vi "CubeDropper.vi"(1 "Shoot":bool, 2 "Height":enum16{"Switch", "Scale", "Bottom", "Null"}(ring)=enum."Scale") -> (0 "CurrentHeight":enum16{"Switch", "Scale", "Bottom", "Null"}(ring))   [LabVIEW 2017]
uses:
  <vilib>/Rock Robotics/WPI/ThirdParty/Phoenix-LabVIEW/Motor Controller/Controls/CTRE_Phoenix_MotorControl_ControlMode.ctl
  <vilib>/Rock Robotics/WPI/ThirdParty/Phoenix-LabVIEW/Motor Controller/Get/CTRE_Phoenix_MotorController_GetQuadratureData.vi
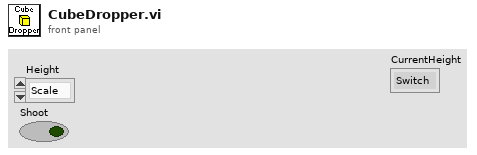
[diagram p1: front panel]
types:
  T1 = typedef "CTRE_Phoenix_MotorControl_ControlMode.ctl" = u16
  T2 = typedef "WPI_MotorControlDeviceRef.ctl" = cluster{"DeviceStatus":errorcluster, "Type":T3, "PWM":cluster{"PWM Channel":T4, "DeadBand":T5}, "CAN":cluster{"Device Number":u8, "SetOutput VI Ref":variant, "GetOutput VI Ref":variant, "Enable VI Ref":variant, "Disable VI Ref":variant, "Data":variant}, "Invert":bool, "DIO PWM":cluster{"PWM \"Enable\" Channel":T4, "DIOChannel":T6, "PWM Rate":dbl}}
  T3 = typedef "WPI_MotorControlType.ctl" = enum16{"PWM", "CAN", "DIO PWM"}
  T4 = typedef "FPGA_DIOPWMChannel.ctl" = enum8{"PWM 0", "PWM 1", "PWM 2", "PWM 3", "PWM 4", "PWM 5", "PWM 6", "PWM 7", "PWM 8", "PWM 9", "PWM MXP 0", "PWM MXP 1", "PWM MXP 2", "PWM MXP 3", "PWM MXP 4", "PWM MXP 5", "PWM MXP 6", "PWM MXP 7", "PWM MXP 8", "PWM MXP 9", "Invalid"}
  T5 = typedef "WPI_PWMDeadband.ctl" = cluster{"Name":string, "maxPositivePwm":i32, "minPositivePwm":i32, "centerPwm":i32, "maxNegativePwm":i32, "minNegativePwm":i32, "angularRange":u16}
  T6 = typedef "FPGA_DIOChannel.ctl" = enum8{"DIO 0", "DIO 1", "DIO 2", "DIO 3", "DIO 4", "DIO 5", "DIO 6", "DIO 7", "DIO 8", "DIO 9", "DIO MXP 0", "DIO MXP 1", "DIO MXP 2", "DIO MXP 3", "DIO MXP 4", "DIO MXP 5", "DIO MXP 6", "DIO MXP 7", "DIO MXP 8", "DIO MXP 9", "DIO MXP 10", "DIO MXP 11", "DIO MXP 12", "DIO MXP 13", "DIO MXP 14", "DIO MXP 15", "SPI Port CS1", "SPI Port CS2", "SPI Port CS3", "SPI Port MISO", "SPI Port MOSI", "Invalid"}
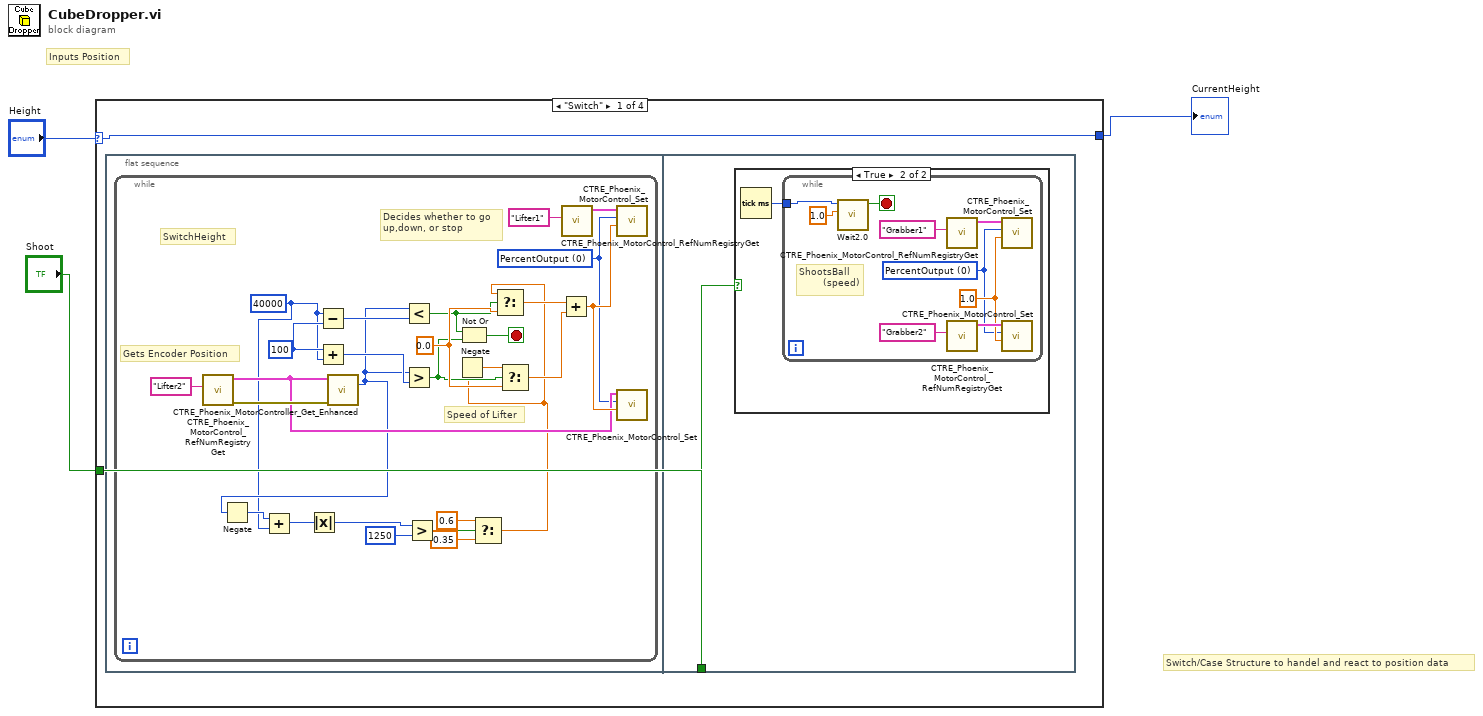
[diagram p0: block diagram]
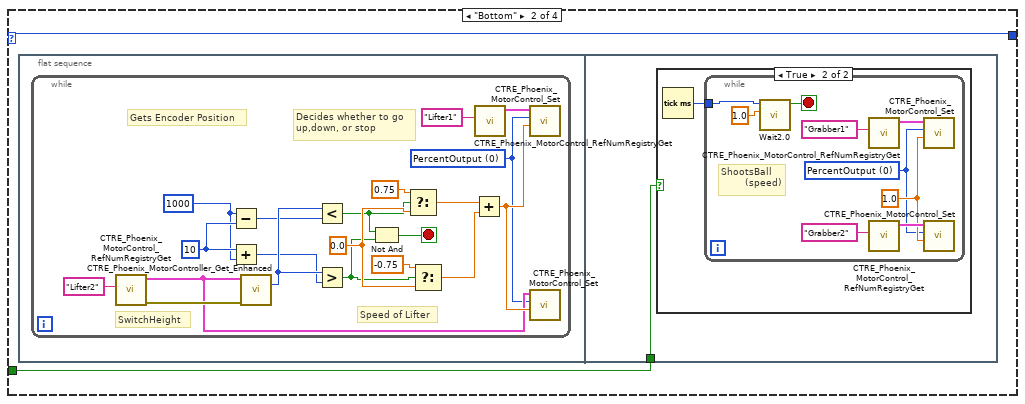
[diagram p3: hidden frame]
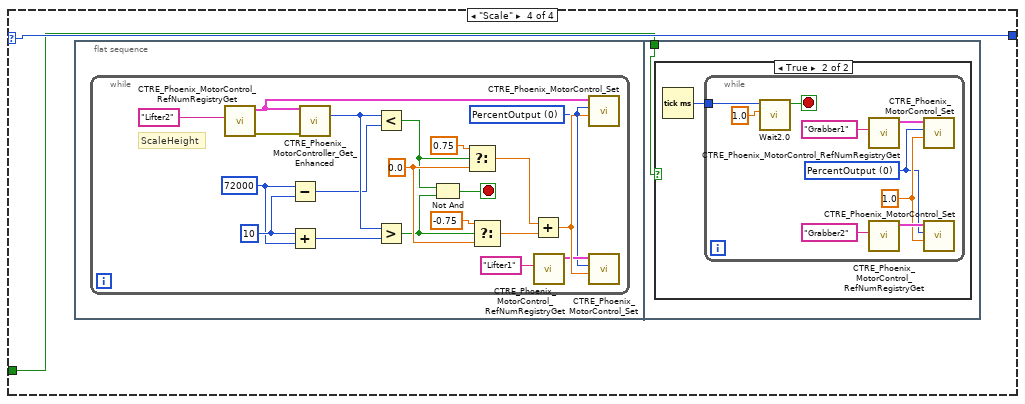
[diagram p6: hidden frame]
diagram:
  # "Switch/Case Structure to handel and react to position data"
  # "Inputs Position"
  n1 = case shown="\"Switch\"" "Height" {
    selector: "Height" -> [w5 w45 w77 w79]
    tunnel: [w5 w45 w77 w79] -> w2
    tunnel: "Shoot" -> [w4 w44 _ w78]
    frame "Switch" {
      n2 = flat-sequence {
        tunnel: w4 -> [w33]
        frame #0 {
          n3 = while {
            stop <- w21 stop-if-true
            w17 = T1 0 items=["PercentOutput"=0, "Position"=1, "Velocity"=2, "Current"=3, "Follower"=5, "MotionProfile"=6, "MotionMagic"=7, "MotionMagicArc"=8, "MotionProfileArc"=10, "Disabled"=15] ("Control Mode")
            w26 = 0.0
            w12 = 40000
            w29 = 100
            # "Speed of Lifter"
            # "Decides whether to go\nup,down, or stop"
            # "Gets Encoder Position"
            # "SwitchHeight"
            n4 = call <vilib>:"CTRE_Phoenix_MotorControl_RefNumRegistryGet.vi"("refnum name"="Lifter2") -> ("error out"=w32:errorcluster, "PhoenixMotorControlDevRef"=w19:T2)  [unwired: 9 in]
            n5 = Subtract(x=w12, y=w29) -> (x-y=w28:i32)
            n6 = Add(x=w29, y=w12) -> (x+y=w27:i32)
            n7 = call-poly <vilib>:"CTRE_Phoenix_MotorController_Get_Enhanced.vi"("PhoenixMotorControlDevRef"=w19, "error in"=w32) -> ("Quadrature Position"=w13:i32)  [unwired: 10 in, 3 out]
            n8 = Negate(x=w13) -> (-x=w14:i32)
            n9 = Add(x=w14, y=w12) -> (x+y=w15:i32)
            n10 = Absolute Value(x=w15) -> (abs(x)=w11:i32)
            n11 = Less?(x=w13, y=w28) -> (x < y?=w23:bool)
            n12 = Greater?(x=w13, y=w27) -> (0:w22:bool)
            n13 = Greater?(x=w11, y=1250) -> (0:w9:bool)
            n14 = Not Or(1:w22, 2:w23) -> (0:w21:bool)
            n15 = Select(t=0.6, s=w9, f=0.35) -> (s? t:f=w6:dbl)
            n16 = Negate(x=w6) -> (-x=w16:dbl)
            n17 = Select(t=w6, s=w23, f=w26) -> (s? t:f=w25:dbl)
            n18 = Select(t=w16, s=w22, f=w26) -> (s? t:f=w24:dbl)
            n19 = Add(x=w25, y=w24) -> (x+y=w20:dbl)
            n20 = call <vilib>:"CTRE_Phoenix_MotorControl_RefNumRegistryGet.vi"("refnum name"="Lifter1") -> ("PhoenixMotorControlDevRef"=w18:T2)  [unwired: 9 in, 1 out]
            n21 = call <vilib>:"CTRE_Phoenix_MotorControl_Set.vi"("Output"=w20, "Control Mode"=w17, "PhoenixMotorControlDevRef"=w18) -> ()  [unwired: 7 in, 2 out]
            n22 = call <vilib>:"CTRE_Phoenix_MotorControl_Set.vi"("Output"=w20, "Control Mode"=w17, "PhoenixMotorControlDevRef"=w19) -> ()  [unwired: 7 in, 2 out]
          }
        }
        frame #1 {
          n23 = case shown="True" w33 {
            frame False {
            }
            frame True {
              n24 = Tick Count (ms)() -> (millisecond timer value=w34:u32)
              n25 = while {
                tunnel: w34 -> [w38]
                stop <- w36 stop-if-true
                w35 = T1 0 items=["PercentOutput"=0, "Position"=1, "Velocity"=2, "Current"=3, "Follower"=5, "MotionProfile"=6, "MotionMagic"=7, "MotionMagicArc"=8, "MotionProfileArc"=10, "Disabled"=15] ("Control Mode")
                w39 = 1.0
                # "ShootsBall\n        (speed)"
                n26 = call "Wait2.0.vi"("Seconds"=1.0, "Start Time"=w38) -> ("Output"=w36:bool)  [unwired: 9 in]
                n27 = call <vilib>:"CTRE_Phoenix_MotorControl_RefNumRegistryGet.vi"("refnum name"="Grabber1") -> ("PhoenixMotorControlDevRef"=w41:T2)  [unwired: 9 in, 1 out]
                n28 = call <vilib>:"CTRE_Phoenix_MotorControl_RefNumRegistryGet.vi"("refnum name"="Grabber2") -> ("PhoenixMotorControlDevRef"=w40:T2)  [unwired: 9 in, 1 out]
                n29 = call <vilib>:"CTRE_Phoenix_MotorControl_Set.vi"("Output"=w39, "Control Mode"=w35, "PhoenixMotorControlDevRef"=w41) -> ()  [unwired: 7 in, 2 out]
                n30 = call <vilib>:"CTRE_Phoenix_MotorControl_Set.vi"("Output"=w39, "Control Mode"=w35, "PhoenixMotorControlDevRef"=w40) -> ()  [unwired: 7 in, 2 out]
              }
            }
          }
        }
      }
    }
    frame "Bottom" {
      n31 = flat-sequence {
        tunnel: w44 -> [w66]
        frame #0 {
          n32 = while {
            stop <- w52 stop-if-true
            w46 = T1 0 items=["PercentOutput"=0, "Position"=1, "Velocity"=2, "Current"=3, "Follower"=5, "MotionProfile"=6, "MotionMagic"=7, "MotionMagicArc"=8, "MotionProfileArc"=10, "Disabled"=15] ("Control Mode")
            w57 = 0.0
            w58 = 1000
            w61 = 10
            # "Speed of Lifter"
            # "Decides whether to go\nup,down, or stop"
            # "Gets Encoder Position"
            # "SwitchHeight"
            n33 = call <vilib>:"CTRE_Phoenix_MotorControl_RefNumRegistryGet.vi"("refnum name"="Lifter2") -> ("error out"=w65:errorcluster, "PhoenixMotorControlDevRef"=w50:T2)  [unwired: 9 in]
            n34 = Subtract(x=w58, y=w61) -> (x-y=w60:i32)
            n35 = Add(x=w61, y=w58) -> (x+y=w59:i32)
            n36 = call-poly <vilib>:"CTRE_Phoenix_MotorController_Get_Enhanced.vi"("PhoenixMotorControlDevRef"=w50, "error in"=w65) -> ("Quadrature Position"=w62:i32)  [unwired: 10 in, 3 out]
            n37 = Less?(x=w62, y=w60) -> (x < y?=w54:bool)
            n38 = Greater?(x=w62, y=w59) -> (0:w53:bool)
            n39 = Not And(1:w53, 2:w54) -> (0:w52:bool)
            n40 = Select(t=0.75, s=w54, f=w57) -> (s? t:f=w56:dbl)
            n41 = Select(t=-0.75, s=w53, f=w57) -> (s? t:f=w55:dbl)
            n42 = Add(x=w56, y=w55) -> (x+y=w51:dbl)
            n43 = call <vilib>:"CTRE_Phoenix_MotorControl_RefNumRegistryGet.vi"("refnum name"="Lifter1") -> ("PhoenixMotorControlDevRef"=w49:T2)  [unwired: 9 in, 1 out]
            n44 = call <vilib>:"CTRE_Phoenix_MotorControl_Set.vi"("Output"=w51, "Control Mode"=w46, "PhoenixMotorControlDevRef"=w49) -> ()  [unwired: 7 in, 2 out]
            n45 = call <vilib>:"CTRE_Phoenix_MotorControl_Set.vi"("Output"=w51, "Control Mode"=w46, "PhoenixMotorControlDevRef"=w50) -> ()  [unwired: 7 in, 2 out]
          }
        }
        frame #1 {
          n46 = case shown="True" w66 {
            frame False {
            }
            frame True {
              n47 = Tick Count (ms)() -> (millisecond timer value=w67:u32)
              n48 = while {
                tunnel: w67 -> [w71]
                stop <- w69 stop-if-true
                w68 = T1 0 items=["PercentOutput"=0, "Position"=1, "Velocity"=2, "Current"=3, "Follower"=5, "MotionProfile"=6, "MotionMagic"=7, "MotionMagicArc"=8, "MotionProfileArc"=10, "Disabled"=15] ("Control Mode")
                w72 = 1.0
                # "ShootsBall\n        (speed)"
                n49 = call "Wait2.0.vi"("Seconds"=1.0, "Start Time"=w71) -> ("Output"=w69:bool)  [unwired: 9 in]
                n50 = call <vilib>:"CTRE_Phoenix_MotorControl_RefNumRegistryGet.vi"("refnum name"="Grabber1") -> ("PhoenixMotorControlDevRef"=w74:T2)  [unwired: 9 in, 1 out]
                n51 = call <vilib>:"CTRE_Phoenix_MotorControl_RefNumRegistryGet.vi"("refnum name"="Grabber2") -> ("PhoenixMotorControlDevRef"=w73:T2)  [unwired: 9 in, 1 out]
                n52 = call <vilib>:"CTRE_Phoenix_MotorControl_Set.vi"("Output"=w72, "Control Mode"=w68, "PhoenixMotorControlDevRef"=w74) -> ()  [unwired: 7 in, 2 out]
                n53 = call <vilib>:"CTRE_Phoenix_MotorControl_Set.vi"("Output"=w72, "Control Mode"=w68, "PhoenixMotorControlDevRef"=w73) -> ()  [unwired: 7 in, 2 out]
              }
            }
          }
        }
      }
    }
    frame "Null", Default {
    }
    frame "Scale" {
      n54 = flat-sequence {
        tunnel: w78 -> [w100]
        frame #0 {
          n55 = while {
            stop <- w86 stop-if-true
            w80 = T1 0 items=["PercentOutput"=0, "Position"=1, "Velocity"=2, "Current"=3, "Follower"=5, "MotionProfile"=6, "MotionMagic"=7, "MotionMagicArc"=8, "MotionProfileArc"=10, "Disabled"=15] ("Control Mode")
            w91 = 0.0
            w92 = 72000
            w95 = 10
            # "ScaleHeight"
            n56 = call <vilib>:"CTRE_Phoenix_MotorControl_RefNumRegistryGet.vi"("refnum name"="Lifter2") -> ("error out"=w99:errorcluster, "PhoenixMotorControlDevRef"=w84:T2)  [unwired: 9 in]
            n57 = Subtract(x=w92, y=w95) -> (x-y=w94:i32)
            n58 = Add(x=w95, y=w92) -> (x+y=w93:i32)
            n59 = call-poly <vilib>:"CTRE_Phoenix_MotorController_Get_Enhanced.vi"("PhoenixMotorControlDevRef"=w84, "error in"=w99) -> ("Quadrature Position"=w96:i32)  [unwired: 10 in, 3 out]
            n60 = Less?(x=w96, y=w94) -> (x < y?=w88:bool)
            n61 = Greater?(x=w96, y=w93) -> (0:w87:bool)
            n62 = Not And(1:w87, 2:w88) -> (0:w86:bool)
            n63 = Select(t=0.75, s=w88, f=w91) -> (s? t:f=w90:dbl)
            n64 = Select(t=-0.75, s=w87, f=w91) -> (s? t:f=w89:dbl)
            n65 = Add(x=w90, y=w89) -> (x+y=w85:dbl)
            n66 = call <vilib>:"CTRE_Phoenix_MotorControl_RefNumRegistryGet.vi"("refnum name"="Lifter1") -> ("PhoenixMotorControlDevRef"=w83:T2)  [unwired: 9 in, 1 out]
            n67 = call <vilib>:"CTRE_Phoenix_MotorControl_Set.vi"("Output"=w85, "Control Mode"=w80, "PhoenixMotorControlDevRef"=w84) -> ()  [unwired: 7 in, 2 out]
            n68 = call <vilib>:"CTRE_Phoenix_MotorControl_Set.vi"("Output"=w85, "Control Mode"=w80, "PhoenixMotorControlDevRef"=w83) -> ()  [unwired: 7 in, 2 out]
          }
        }
        frame #1 {
          n69 = case shown="True" w100 {
            frame False {
            }
            frame True {
              n70 = Tick Count (ms)() -> (millisecond timer value=w101:u32)
              n71 = while {
                tunnel: w101 -> [w105]
                stop <- w103 stop-if-true
                w102 = T1 0 items=["PercentOutput"=0, "Position"=1, "Velocity"=2, "Current"=3, "Follower"=5, "MotionProfile"=6, "MotionMagic"=7, "MotionMagicArc"=8, "MotionProfileArc"=10, "Disabled"=15] ("Control Mode")
                w106 = 1.0
                n72 = call "Wait2.0.vi"("Seconds"=1.0, "Start Time"=w105) -> ("Output"=w103:bool)  [unwired: 9 in]
                n73 = call <vilib>:"CTRE_Phoenix_MotorControl_RefNumRegistryGet.vi"("refnum name"="Grabber1") -> ("PhoenixMotorControlDevRef"=w108:T2)  [unwired: 9 in, 1 out]
                n74 = call <vilib>:"CTRE_Phoenix_MotorControl_RefNumRegistryGet.vi"("refnum name"="Grabber2") -> ("PhoenixMotorControlDevRef"=w107:T2)  [unwired: 9 in, 1 out]
                n75 = call <vilib>:"CTRE_Phoenix_MotorControl_Set.vi"("Output"=w106, "Control Mode"=w102, "PhoenixMotorControlDevRef"=w108) -> ()  [unwired: 7 in, 2 out]
                n76 = call <vilib>:"CTRE_Phoenix_MotorControl_Set.vi"("Output"=w106, "Control Mode"=w102, "PhoenixMotorControlDevRef"=w107) -> ()  [unwired: 7 in, 2 out]
              }
            }
          }
        }
      }
    }
  }
  "CurrentHeight" <- w2
